vi "imaq set keys.vi"(8 "error in (no error)":errorcluster, 9 "Array":string[](array[string]), 10 "Keys":string[](array[string]), 11 "Refnum in":T1) -> (0 "error out":errorcluster, 3 "Refnum out":T1)   [LabVIEW 2020, in "Point Grey Camera.lvclass"]
uses:
  Point Grey Camera.lvclass
  IMAQ Image.ctl
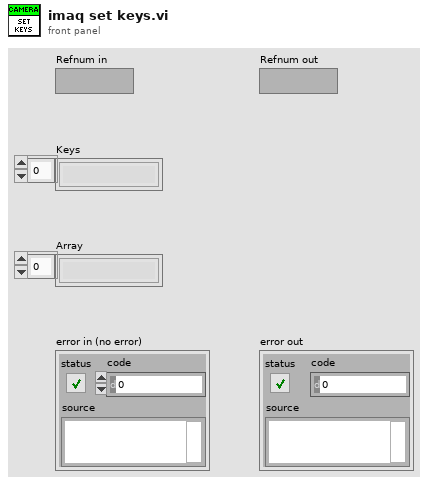
[diagram p1: front panel]
types:
  T1 = typedef "IMAQ Image.ctl" = refnum<image>
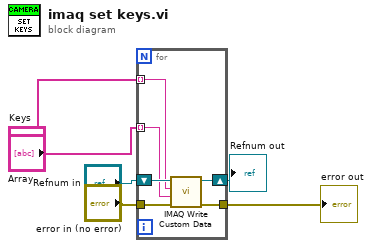
[diagram p0: block diagram]
diagram:
  n1 = for {
    shift-right: [w11] -> w2
    shift-left: "Refnum in" -> [w12]
    tunnel: "Keys" -> [w9] mode=indexing
    tunnel: "Array" -> [w10] mode=indexing
    tunnel: "error in (no error)" -> [w8]
    tunnel: [w7] -> w6
    n2 = call "IMAQ Write Custom Data"("error in (no error)"=w8, "Custom Data In"=w10, "Key"=w9, "Image"=w12) -> ("error out"=w7:errorcluster, "Image Out"=w11:T1)  [unwired: 6 in]
  }
  "error out" <- w6
  "Refnum out" <- w2
